vi "Axis Scale F.vi"(7 "Enum":enum16{"Initial", "Read"}(ring)=enum."Read", 8 "error In":errorcluster, 11 "Axis":i32) -> (0 "error Out":errorcluster, 2 "Scale":dbl)   [LabVIEW 2019]
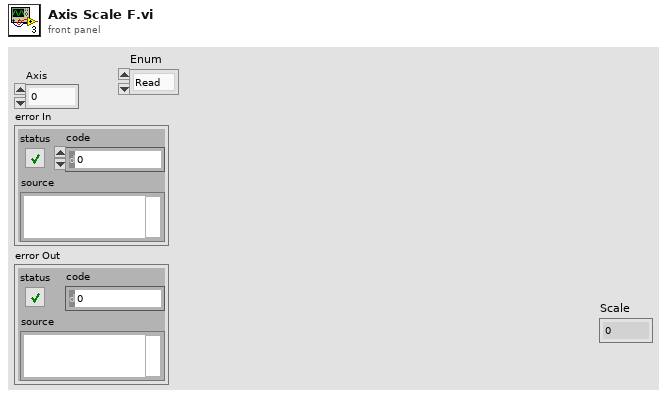
[diagram p1: front panel]
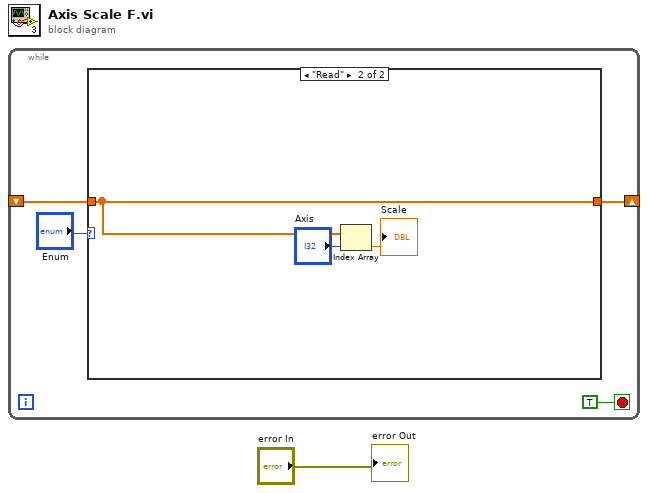
[diagram p0: block diagram]
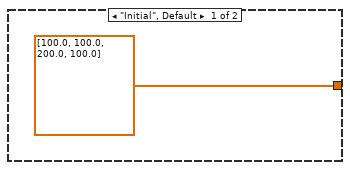
[diagram p2: hidden frame]
diagram:
  n1 = while {
    shift-right: [w4] -> _
    shift-left: _ -> [w3]
    stop <- TRUE stop-if-true
    n2 = case shown="\"Read\"" "Enum" {
      tunnel: [dbl[] [100.0, 100.0, 200.0, 100.0] w9] -> w4
      tunnel: w3 -> [_ w9]
      frame "Initial", Default {
      }
      frame "Read" {
        n3 = Index Array(array=w9, index="Axis") -> (element=→"Scale":dbl)
      }
    }
  }
  "error Out" <- "error In"
